vi "checkChecksum.vi"(8 "error in (no error)":errorcluster, 10 "TPDO data":u8[](array[numeric]), 11 "OrionBMS in":refnum<class "OrionBMSClass.lvclass">) -> (0 "error in (no error) 2":errorcluster, 2 "checkSumMatched":bool, 3 "OrionBMS out":refnum<class "OrionBMSClass.lvclass">)   [LabVIEW 2018, in "OrionBMSClass.lvclass"]
uses:
  OrionBMSClass.lvclass
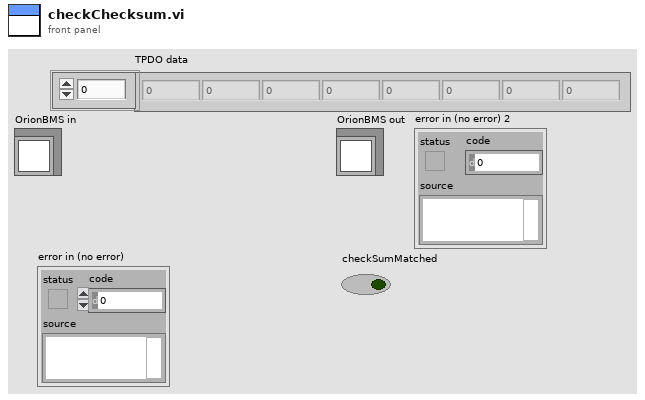
[diagram p1: front panel]
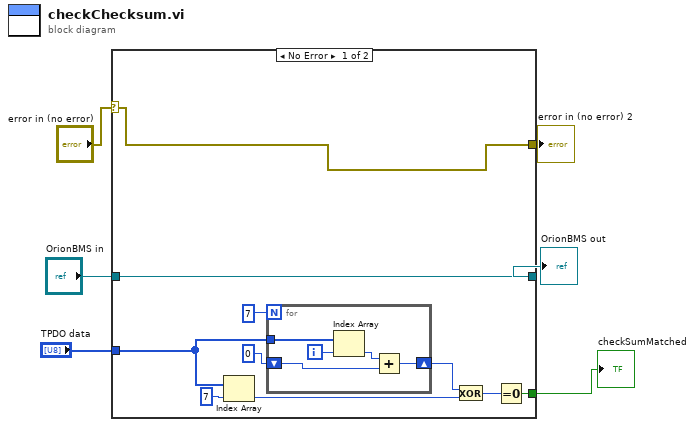
[diagram p0: block diagram]
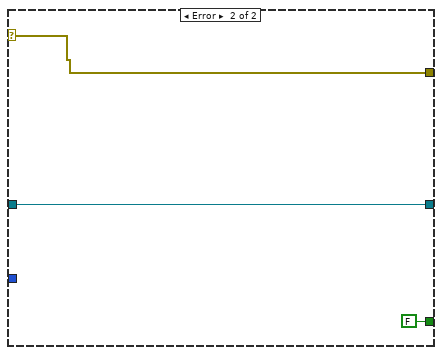
[diagram p2: hidden frame]
diagram:
  n1 = case shown="No Error" "error in (no error)" {
    selector: "error in (no error)" -> [w7 w22]
    tunnel: [w16 w24] -> w6
    tunnel: "OrionBMS in" -> [w16 w24]
    tunnel: "TPDO data" -> [w9 _]
    tunnel: [w8 FALSE] -> w3
    tunnel: [w7 w22] -> w2
    frame No Error {
      n2 = Index Array(array=w9, index=7) -> (element=w14:u8)
      n3 = for {
        N: 7 -> [_]
        tunnel: w9 -> [w21]
        shift-right: [w18] -> w10
        shift-left: u8 0 -> [w17]
        i -> [w20]
        n4 = Index Array(array=w21, index=w20) -> (element=w19:u8)
        n5 = Add(x=w19, y=w17) -> (x+y=w18:u8)
      }
      n6 = Exclusive Or(1:w14, 2:w10) -> (0:w11:u8)
      n7 = Equal To 0?(x=w11) -> (x = 0?=w8:bool)
    }
    frame Error {
    }
  }
  "OrionBMS out" <- w6
  "error in (no error) 2" <- w2
  "checkSumMatched" <- w3
